vi "Gear_Ratio_to_Counts.vi"(4 "theta 4":dbl, 5 "theta 3":dbl, 6 "theta 2":dbl, 7 "theta 1":dbl) -> (0 "j4":i32, 1 "j3":i32, 2 "j2":i32, 3 "j1":i32)   [LabVIEW 2016]
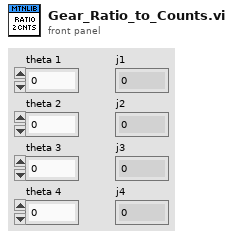
[diagram p1: front panel]
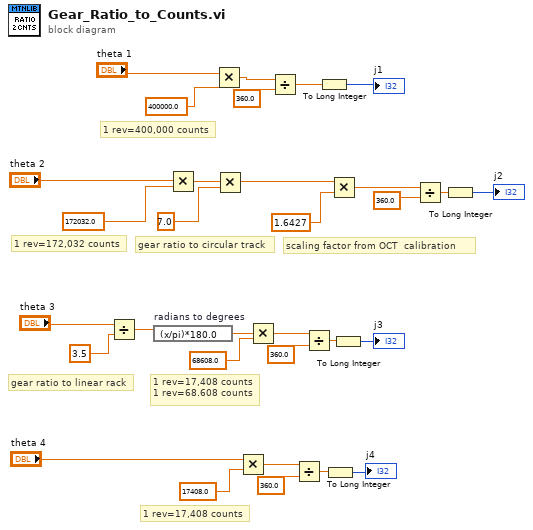
[diagram p0: block diagram]
diagram:
  # "scaling factor from OCT  calibration"
  # "1 rev=17,408 counts"
  # "1 rev=17,408 counts\n1 rev=68.608 counts"
  # "gear ratio to linear rack"
  # "gear ratio to circular track"
  # "1 rev=172,032 counts"
  # "1 rev=400,000 counts"
  n1 = Divide(x="theta 3", y=3.5) -> (x/y=w25:dbl)
  n2 = expression code="(x/pi)*180.0" "radians to degrees"(w25) -> (w23:dbl)
  n3 = Multiply(x="theta 2", y=172032.0) -> (x*y=w20:dbl)
  n4 = Multiply(x="theta 1", y=400000.0) -> (x*y=w31:dbl)
  n5 = Multiply(x=w20, y=7.0) -> (x*y=w3:dbl)
  n6 = Multiply(x="theta 4", y=17408.0) -> (x*y=w15:dbl)
  n7 = Multiply(x=w23, y=68608.0) -> (x*y=w21:dbl)
  n8 = Divide(x=w31, y=360.0) -> (x/y=w11:dbl)
  n9 = Divide(x=w15, y=360.0) -> (x/y=w5:dbl)
  n10 = Divide(x=w21, y=360.0) -> (x/y=w7:dbl)
  n11 = To Long Integer(number=w11) -> (32bit integer=→"j1":i32)
  n12 = To Long Integer(number=w5) -> (32bit integer=→"j4":i32)
  n13 = Multiply(x=w3, y=1.6427) -> (x*y=w2:dbl)
  n14 = To Long Integer(number=w7) -> (32bit integer=→"j3":i32)
  n15 = Divide(x=w2, y=360.0) -> (x/y=w9:dbl)
  n16 = To Long Integer(number=w9) -> (32bit integer=→"j2":i32)
